vi "Control measurement.vi"(0 "CV configuration":T2={"E begin (V)"=0.0, "E vertex 1 (V)"=0.0, "E vertex 2 (V)"=0.0, "Cycles"=1, "Scan rate (V/s)"=0.01, "E step (V)"=0.01} {"E step (V)" min=0.01 max=0.25; "Scan rate (V/s)" min=0.01 max=10.0; "Cycles" min=1; "E vertex 2 (V)" min=-3.3 max=3.3; "E vertex 1 (V)" min=-3.3 max=3.3; "E begin (V)" min=-3.3 max=3.3}, 1 "App state":T1, 3 "Error in":errorcluster) -> (5 "App state":T1, 7 "Error out":errorcluster)   [LabVIEW 2021]
uses:
  Typedefs/State.ctl
  Typedefs/CV configuration.ctl
  Global variables/VISA resource.vi
  COBS/COBS.lvlib
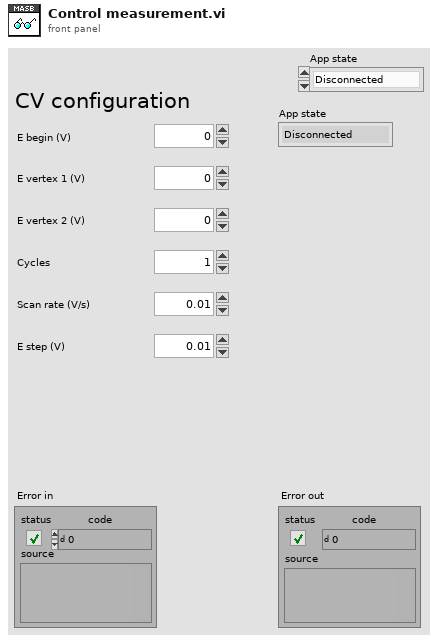
[diagram p1: front panel]
types:
  T1 = typedef "State.ctl" = enum16{"Disconnected", "Connected", "Measuring"}
  T2 = typedef "CV configuration.ctl" = cluster{"E begin (V)":dbl, "E vertex 1 (V)":dbl, "E vertex 2 (V)":dbl, "Cycles":u8, "Scan rate (V/s)":dbl, "E step (V)":dbl}
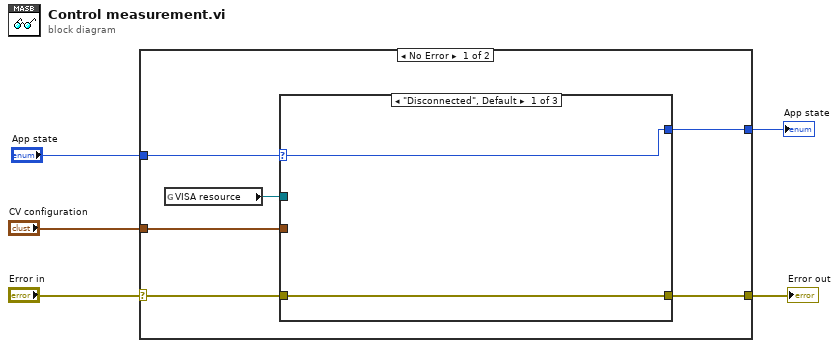
[diagram p0: block diagram]
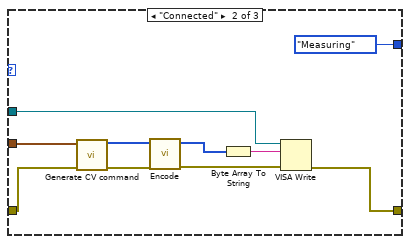
[diagram p2: hidden frame]
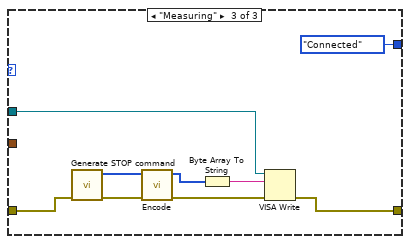
[diagram p3: hidden frame]
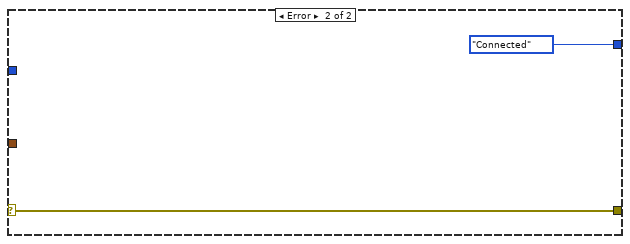
[diagram p4: hidden frame]
diagram:
  n1 = case shown="No Error" "Error in" {
    selector: "Error in" -> [w10 w34]
    tunnel: [w8 w34] -> w4
    tunnel: [w11 State."Connected" ("App state")] -> w3
    tunnel: "CV configuration" -> [w9 _]
    tunnel: "App state" -> [w6 _]
    frame No Error {
      n2 = global read "VISA resource.vi" "VISA resource"() -> (w7:refnum<visa-resource-name>)
      n3 = case shown="\"Disconnected\", Default" w6 {
        selector: w6 -> [w13 _ _]
        tunnel: [w13 State."Measuring" ("App state") State."Connected" ("App state")] -> w11
        tunnel: w10 -> [w12 w22 w28]
        tunnel: w9 -> [_ w21 _]
        tunnel: [w12 w19 w30] -> w8
        tunnel: w7 -> [_ w18 w29]
        frame "Disconnected", Default {
        }
        frame "Connected" {
          n4 = call "Generate CV command.vi"("Error in"=w22, "CV configuration"=w21) -> ("Error out"=w17:errorcluster, "Paquet command"=w14:u8[])  [unwired: 8 in]
          n5 = call "Encode.vi"("Error in"=w17, "Decoded message"=w14) -> ("Error out"=w16:errorcluster, "Encoded message"=w15:u8[])  [unwired: 8 in]
          n6 = Byte Array To String(unsigned byte array=w15) -> (string=w20:string)
          n7 = VISA Write(VISA resource name=w18, write buffer=w20, error in (no error)=w16) -> (error out=w19:errorcluster)  [unwired: 2 out]
        }
        frame "Measuring" {
          n8 = call "Generate STOP command.vi"("Error in"=w28) -> ("Error out"=w26:errorcluster, "Array"=w25:u8[])  [unwired: 9 in]
          n9 = call "Encode.vi"("Error in"=w26, "Decoded message"=w25) -> ("Error out"=w27:errorcluster, "Encoded message"=w24:u8[])  [unwired: 8 in]
          n10 = Byte Array To String(unsigned byte array=w24) -> (string=w31:string)
          n11 = VISA Write(VISA resource name=w29, write buffer=w31, error in (no error)=w27) -> (error out=w30:errorcluster)  [unwired: 2 out]
        }
      }
    }
    frame Error {
    }
  }
  "Error out" <- w4
  "App state" <- w3
